vi "例10.4  利用高层函数采集N幅图像（sequence）.vi"() -> ()   [LabVIEW 2012]
doc: "The Sequence VI acquires a sequence of images and displays the images in an image control using high-level acquisition VIs. A sequence is appropriate for applications in which you want to process multiple images."
uses:
  <vilib>/userdefined/High Color/IMAQdx.ctl
  <vilib>/vision/driver/NI_Vision_Acquisition_Software.lvlib
panel:
  in  "Camera Name":T1
  out "Image Array":T2[](array[plugin-control])
  in  "Number of Images":i32=5
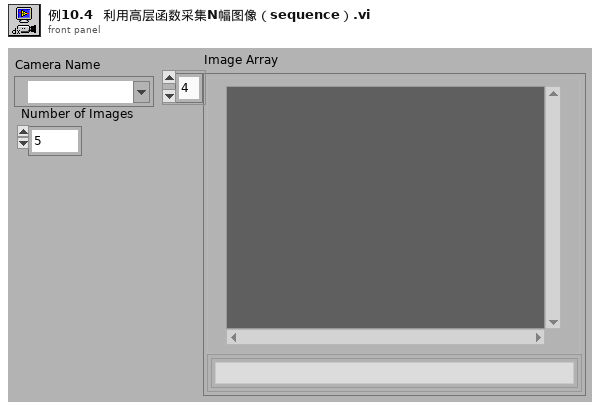
[diagram p1: front panel]
types:
  T1 = typedef "IMAQdx.ctl" = refnum<k21>
  T2 = typedef "IMAQ Image.ctl" = refnum<image>
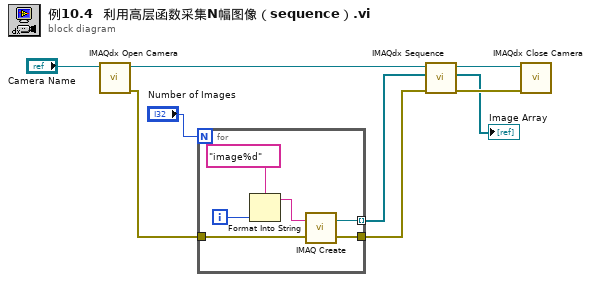
[diagram p0: block diagram]
diagram:
  n1 = call <vilib>:"IMAQdx Open Camera.vi"("Session In"="Camera Name") -> ("error out"=w8:errorcluster, "Session Out"=w4:T1)  [unwired: 2 in, 7 out]
  n2 = for {
    N: "Number of Images" -> [_]
    tunnel: w8 -> [w15]
    tunnel: [w14] -> w6 mode=indexing
    tunnel: [w13] -> w7
    i -> [w12]
    n3 = Format Into String(format string="image%d" ("Image Name"), w12) -> (resulting string=w11:string)  [unwired: 2 in, 1 out]
    n4 = call "IMAQ Create"("Image Name"=w11, "error in (no error)"=w15) -> ("New Image"=w14:T2, "error out"=w13:errorcluster)  [unwired: 2 in, 1 out]
  }
  n5 = call <vilib>:"IMAQdx Sequence.vi"("error in"=w7, "Images In"=w6, "Session In"=w4) -> ("error out"=w5:errorcluster, "Images Out"=→"Image Array":T2[], "Session Out"=w1:T1)  [unwired: 6 out]
  n6 = call <vilib>:"IMAQdx Close Camera.vi"("error in"=w5, "Session In"=w1) -> ()  [unwired: 10 out]
